vi "StatisticalData.vi"(0 "configuration file path":path caption="配置文件的路径", 5 "error in (no error)":errorcluster caption="错误输入（无错误）") -> (15 "字符串数组":string[](array[string]), 16 "双精度数组":dbl[](array[numeric]), 19 "error out":errorcluster caption="错误输出")   [LabVIEW 2018]
uses:
  <vilib>/Utility/config.llb/Read Key (Double).vi
  <vilib>/Utility/config.llb/NI_LVConfig.lvlib
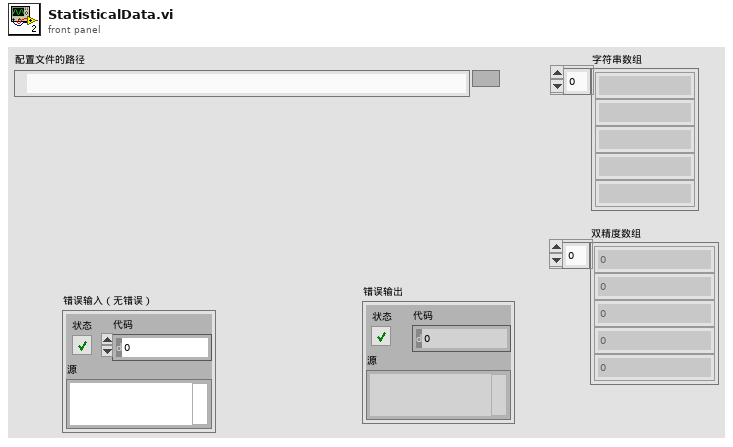
[diagram p1: front panel]
types:
  T1 = typedef "NI_LVConfig.lvlib/Config Data RefNum.ctl" = refnum<k1>
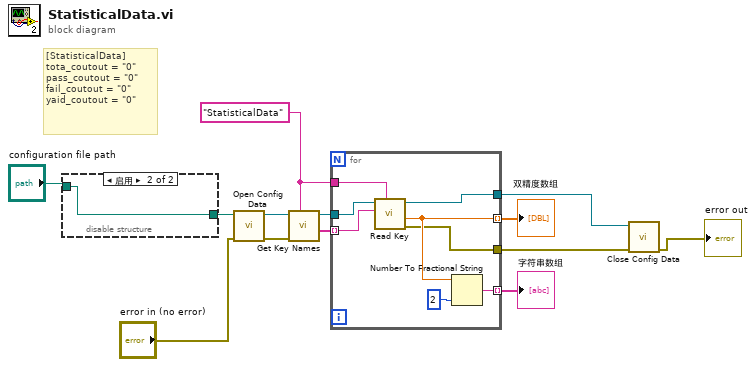
[diagram p0: block diagram]
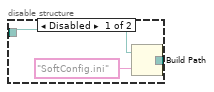
[diagram p2: hidden frame]
diagram:
  w11 = "StatisticalData" ("section")
  # "[StatisticalData]\ntota_coutout = \"0\"\npass_coutout = \"0\"\nfail_coutout = \"0\"\nyaid_coutout = \"0\""
  n1 = disable-structure shown="启用" {
    disable-tunnel: "configuration file path" -> [w15 w17]
    disable-tunnel: [w14 w17] -> w6
    frame Disabled {
      n2 = Build Path(base path=w15, name or relative path="SoftConfig.ini" ("名称或相对路径")) -> (appended path=w14:path)
    }
    frame Enabled {
    }
  }
  n3 = call <vilib>:"Open Config Data.vi"("error in (no error)"="error in (no error)", "configuration file path"=w6) -> ("error out"=w2:errorcluster, "refnum"=w13:T1)  [unwired: 7 in, 1 out]
  n4 = call <vilib>:"Get Key Names.vi"("section"=w11, "error in (no error)"=w2, "refnum"=w13) -> ("key names"=w12:string[], "refnum out"=w10:T1)  [unwired: 5 in, 2 out]
  n5 = for {
    tunnel: w12 -> [w24] mode=indexing
    tunnel: w11 -> [w25]
    tunnel: w10 -> [w23]
    tunnel: [w22] -> w9 mode=indexing
    tunnel: [w20] -> w8 mode=indexing
    tunnel: [w19] -> w5
    tunnel: [w18] -> w4
    n6 = call-poly <vilib>:"Read Key.vi"("section"=w25, "key"=w24, "refnum"=w23) -> ("error out"=w18:errorcluster, "value"=w22:dbl, "refnum out"=w19:T1)  [unwired: 5 in, 1 out]
    n7 = Number To Fractional String(number=w22, precision (6)=i16 2 ("精度(6)")) -> (F-format string=w20:string)  [unwired: 2 in]
  }
  "字符串数组" <- w8
  "双精度数组" <- w9
  n8 = call <vilib>:"Close Config Data.vi"("error in (no error)"=w4, "refnum"=w5) -> ("error out"=→"error out":errorcluster)  [unwired: 8 in, 1 out]
